vi "create.SequencedUnitHeader.vi"(11 "SequencedUnitHeader.Parms":T1={"Hdr Count"=0, "Hdr Unit"=1, "Hdr Sequence"=1, "Starting Sequence"=1}) -> (2 "Bytes.Out":u8[](array[numeric])=[8, 0, 0, 1, 1, 0, 0, 0] format="%.0x", 3 "PitchMessage out":refnum<class "SequencedUnitHeader.lvclass">)   [LabVIEW 2020]
uses:
  SequencedUnitHeader/SequencedUnitHeader.lvclass
  SequencedUnitHeader/SequencedUnitHeader.Parameters.ctl
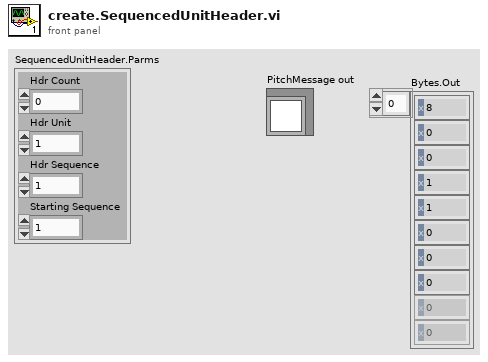
[diagram p1: front panel]
types:
  T1 = typedef "SequencedUnitHeader.lvclass/SequencedUnitHeader.Parameters.ctl" = cluster{"Hdr Count":u8, "Hdr Unit":u8, "Hdr Sequence":u32, "Starting Sequence":u32}
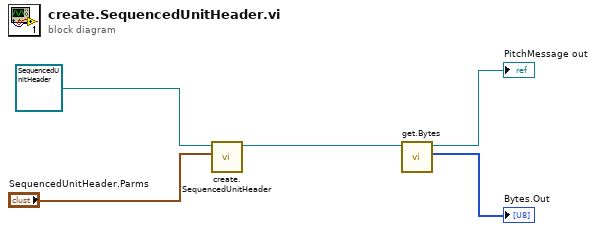
[diagram p0: block diagram]
diagram:
  n1 = call-dynamic "create.SequencedUnitHeader.vi"("SequencedUnitHeader.Parms"="SequencedUnitHeader.Parms", "SequencedUnitHeader in"=refnum<class "SequencedUnitHeader.lvclass"> refnum ("SequencedUnitHeader.lvclass")) -> ("SequencedUnitHeader out"=w4:refnum<class "SequencedUnitHeader.lvclass">)  [unwired: 8 in, 1 out]
  n2 = call-dynamic "get.Bytes.vi"("SequencedUnitHeader in"=w4) -> ("Bytes.Out"=→"Bytes.Out":u8[], "SequencedUnitHeader out"=→"PitchMessage out":refnum<class "SequencedUnitHeader.lvclass">)  [unwired: 8 in, 1 out]
